vi "test图层(1)-修改乱七八糟.vi"() -> ()   [LabVIEW 2018]
doc: "This example demonstrates the use of binary morphological reconstruction in the particle analysis. The example allows you to keep the particles completely inside the ROI, completely outside the ROI or on the ROI."
panel:
  out "Image 2":T1(plugin-control)
  out "框&图层计数":dbl
  in  "Stop":bool
  in  "Operation":enum16{"overlay rectangle"}(ring)
  out "Reconstructed Image":T1(plugin-control)
  out "Image":T1(plugin-control)
  out "框&图层计数 2":dbl
  # "Overview: Demonstrate the use of the Binary Morphology Reconstruction feature of Vision Development Module.\nRequirements: Vision Development Module.\nInstructions:\n1. Run the VI.\n2. Select the ROI in which you want to filter the objects. Press the <Ctrl> key to select multiple ROIs. \n3. Choose the required \"Operation\".\n  - Inner particles: Keeps all the particles completely inside the ROI.\n  - Outer particles: Keeps the particles completely outside the ROI.\n  - Boundary particles: Keeps the particles which are touching the boundary."
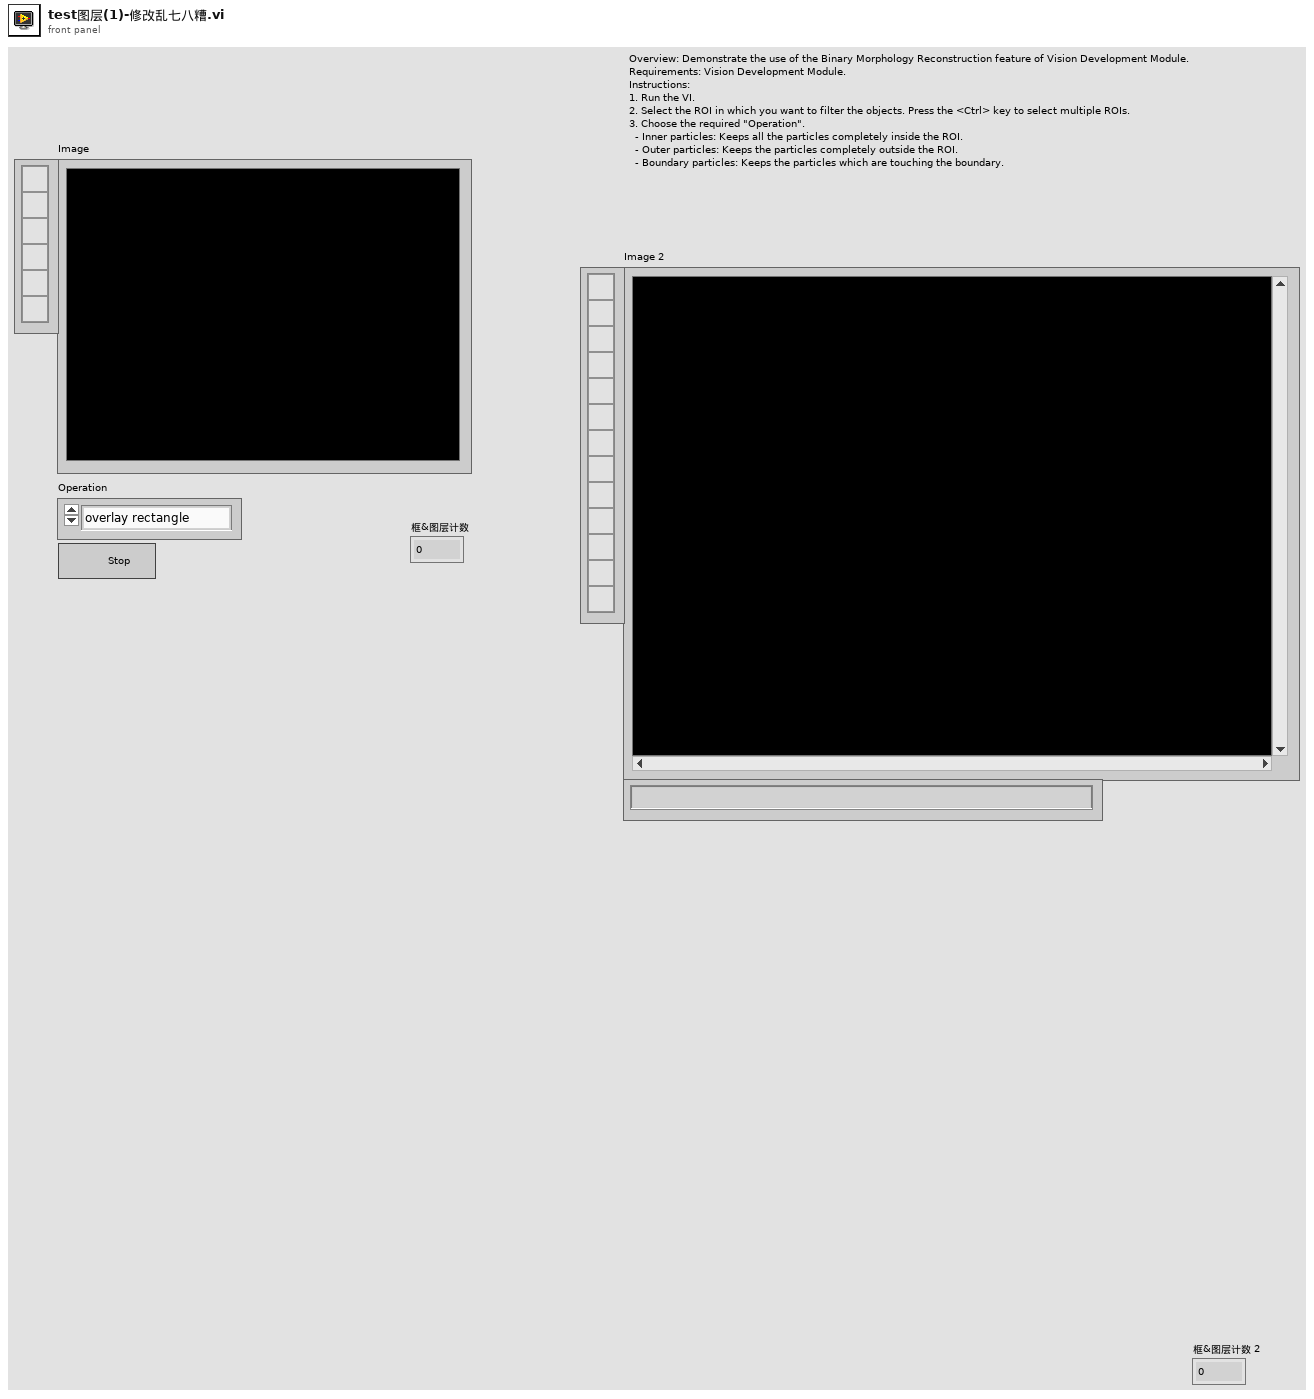
[diagram p1: front panel]
types:
  T1 = typedef "IMAQ Image.ctl" = refnum<image>
  T2 = typedef "Image Type" = u32
  T3 = cluster{"Global Rectangle":i32[], "Contours":cluster{"Contour Type":u32, "ROI Type":u32, "Points":i32[]}[]}
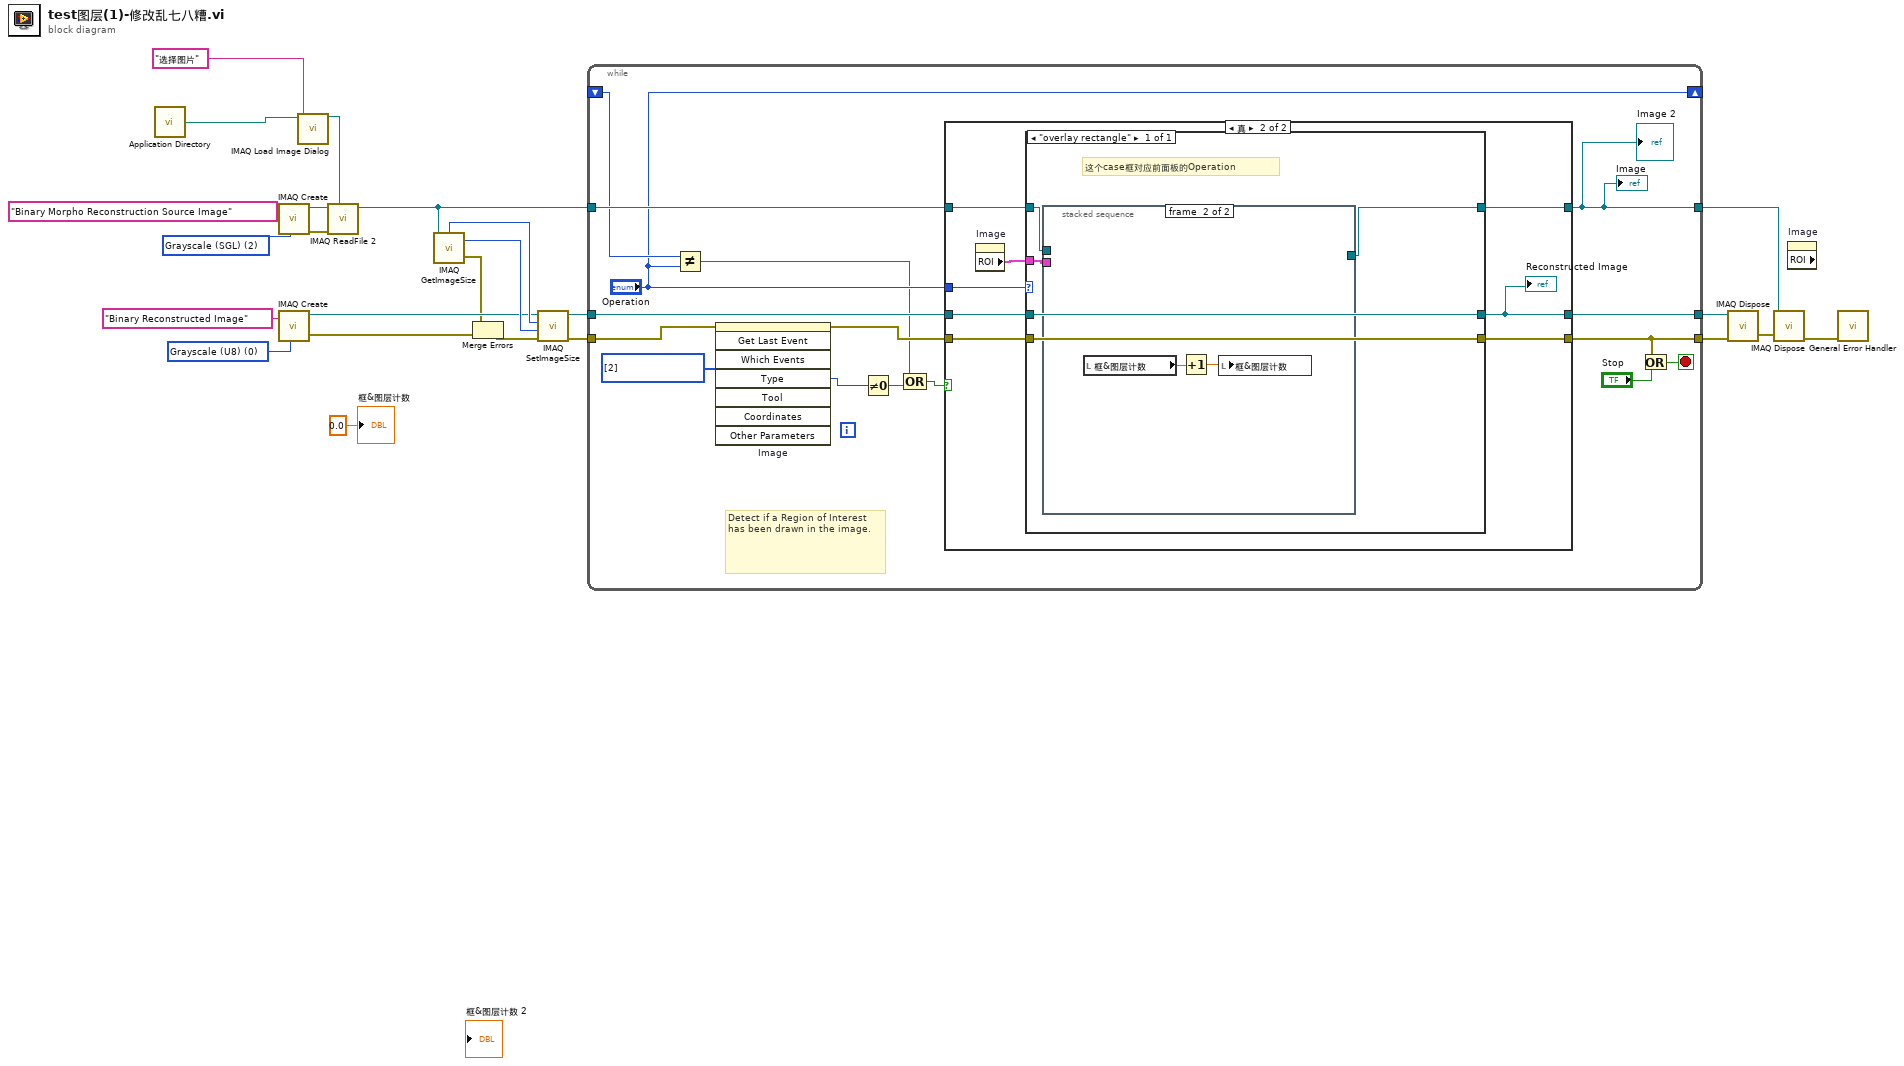
[diagram p0: block diagram]
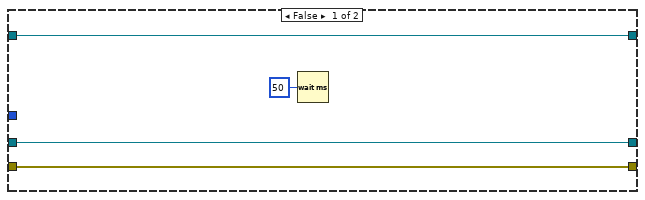
[diagram p2: hidden frame]
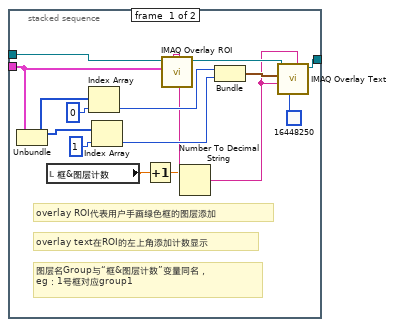
[diagram p3: hidden frame]
diagram:
  w2 = T2 2 items=["Grayscale (U8)", "Grayscale (I16)", "Grayscale (SGL)", "Complex (CSG)", "RGB (U32)", "HSL (U32)", "RGB (U64)", "Grayscale (U16)"] ("Image Type")
  w17 = T2 0 items=["Grayscale (U8)", "Grayscale (I16)", "Grayscale (SGL)", "Complex (CSG)", "RGB (U32)", "HSL (U32)", "RGB (U64)", "Grayscale (U16)"] ("Image Type")
  n1 = call <vilib>:"Application Directory.vi"() -> ("Application Directory"=w24:path)
  n2 = call "IMAQ Create"("Image Name"="Binary Morpho Reconstruction Source Image", "Image Type"=w2) -> ("New Image"=w20:T1, "error out"=w12:errorcluster)  [unwired: 2 in, 1 out]
  n3 = call "IMAQ Create"("Image Name"="Binary Reconstructed Image", "Image Type"=w17) -> ("New Image"=w14:T1, "error out"=w11:errorcluster)  [unwired: 2 in, 1 out]
  n4 = call "IMAQ Load Image Dialog"("Prompt"="选择图片", "Start Path"=w24) -> ("Path"=w3:path)  [unwired: 7 in, 2 out]
  n5 = call "IMAQ ReadFile 2"("File Path"=w3, "error in (no error)"=w12, "Image"=w20) -> ("Image Out"=w4:T1)  [unwired: 4 in, 4 out]
  n6 = call "IMAQ GetImageSize"("Image"=w4) -> ("Y Resolution"=w15:i32, "X Resolution"=w16:i32, "error out"=w8:errorcluster)  [unwired: 1 in, 2 out]
  n7 = Merge Errors(w8, w11) -> (w10:errorcluster)
  n8 = call "IMAQ SetImageSize"("error in (no error)"=w10, "Y Resolution"=w15, "X Resolution"=w16, "Image"=w14) -> ("error out"=w9:errorcluster, "Image Out"=w13:T1)  [unwired: 1 out]
  n9 = while {
    tunnel: w4 -> [w40]
    tunnel: w13 -> [w39]
    tunnel: [w38] -> w19
    tunnel: [w25] -> w18
    shift-right: ["Operation"] -> _
    shift-left: _ -> [w37]
    tunnel: w9 -> [w33]
    tunnel: [w28] -> w7
    stop <- w26 stop-if-true
    w34 = i32[] [2] items=["No Event"=0, "Click Event"=1, "Draw Event"=2, "Size Event"=4, "Scroll Event"=5, "Double Click Event"=8] ("Which Events")
    # "Detect if a Region of Interest has been drawn in the image."
    n10 = Not Equal?(x=w37, y="Operation") -> (x != y?=w31:bool)
    n11 = invoke on="Image" class="ImageControl" method="Get Last Event"(error in=w33, "Which Events"=w34) -> (error out=w32:errorcluster, "Type"=w35:i32)  [unwired: 6 in, 6 out]
    n12 = Not Equal To 0?(x=w35) -> (x != 0?=w30:bool)
    n13 = Compound Arithmetic op=OR(w31, w30) -> (w29:bool)
    n14 = case shown="真" w29 {
      tunnel: w40 -> [w44 w52]
      tunnel: w39 -> [w43 w51]
      tunnel: [w43 w50] -> w38
      tunnel: [w44 w49] -> w25
      tunnel: "Operation" -> [_ w47]
      tunnel: w32 -> [w42 w46]
      tunnel: [w42 w45] -> w28
      frame False {
        n15 = Wait (ms)(milliseconds to wait=u32 50) -> ()  [unwired: 1 out]
      }
      frame True {
        n16 = property on="Image" class="ImageControl"() -> ("ROI"=w48:T3)  [unwired: 2 in, 2 out]
        n17 = case shown="\"overlay rectangle\"" w47 {
          tunnel: w52 -> [w55]
          tunnel: w51 -> [w57]
          tunnel: [w57] -> w50
          tunnel: w48 -> [w53]
          tunnel: [w54] -> w49
          tunnel: w46 -> [w56]
          tunnel: [w56] -> w45
          frame "overlay rectangle" {
            # "这个case框对应前面板的Operation"
            n18 = stacked-sequence {
              tunnel: w55 -> [w71 _]
              tunnel: [w69 _] -> w54
              tunnel: w53 -> [w68 _]
              frame #0 {
                # "图层名Group与“框&图层计数”变量同名，\neg：1号框对应group1"
                # "overlay text在ROI的左上角添加计数显示"
                # "overlay ROI代表用户手画绿色框的图层添加"
                n19 = Unbundle(w68) -> ("Global Rectangle"=w65:i32[])  [unwired: 1 out]
                n20 = local read "框&图层计数"() -> (w60:dbl)
                n21 = Index Array(array=w65, index=0 ("索引")) -> (element=w64:i32)
                n22 = Index Array(array=w65, index=1 ("索引")) -> (element=w63:i32)
                n23 = Increment(x=w60) -> (x+1=w58:dbl)
                n24 = Number To Decimal String(number=w58) -> (decimal integer string=w59:string)  [unwired: 1 in]
                n25 = call "IMAQ Overlay ROI"("Group"=w59, "ROI Descriptor"=w68, "Image"=w71) -> ("Image Out"=w70:T1)  [unwired: 7 in, 1 out]
                n26 = Bundle(w64, w63) -> (w62:cluster{i32, i32})  [unwired: 1 in]
                n27 = call "IMAQ Overlay Text"("Group"=w59, "Text Color (black)"=u32 16448250, "String"=w59, "Origin"=w62, "Image"=w70) -> ("Image Out"=w69:T1)  [unwired: 5 in, 1 out]
              }
              frame #1 {
                n28 = local read "框&图层计数"() -> (w73:dbl)
                n29 = Increment(x=w73) -> (x+1=w72:dbl)
                n30 = local write "框&图层计数"(w72) -> ()
              }
            }
          }
        }
        "Reconstructed Image" <- w50
      }
    }
    "Image" <- w25
    "Image 2" <- w25
    n31 = Or(x=w28, y="Stop") -> (x .or. y?=w26:bool)
  }
  n32 = call "IMAQ Dispose"("Image"=w19, "error in (no error)"=w7) -> ("error out"=w6:errorcluster)  [unwired: 1 in, 3 out]
  n33 = call "IMAQ Dispose"("Image"=w18, "error in (no error)"=w6) -> ("error out"=w1:errorcluster)  [unwired: 1 in, 3 out]
  n34 = property on="Image" class="ImageControl" props=["ROI"]() -> ()  [unwired: 2 in, 3 out]
  n35 = call <vilib>:"General Error Handler.vi"("error in (no error)"=w1) -> ()  [unwired: 10 in, 5 out]
  "框&图层计数" <- 0.0 ("数值")
